vi "Initialize FakedArray.vi"(4 "User events":T8, 6 "Color":T7=9868950, 7 "ToMoreSpecific":T9, 8 "error in (no error)":errorcluster, 9 "Data":T10, 10 "Cluster Refnum":refnum<vi>, 11 "Data in":T1={"Class"={"Ants"=refnum, "Layer"=refnum, "Templates"=refnum, "Icon"=refnum, "Glyph"=refnum, "Settings"=refnum, "Tools"=refnum}, "Ref"={"Add Layer"=refnum, "Remove Layer"=refnum, "Line Text"=[], "Body Text Spec"=refnum, "DNL_Font"=refnum, "glyph path str"=refnum, "templates path str"=refnum, "Arrow Up"=refnum, "Arrow Down"=refnum, "IE VI Ref"=refnum, "Glyphs tree"=refnum, "Templates tree"=refnum, "Layer Icon Text"=refnum, "Layer Template"=refnum, "Clipboard"=refnum, "BW icon in"=refnum, "Color icon in"=refnum, "Layer Clust"=refnum, "Body Text"=refnum, "DNL_Framework Templates"=refnum, "Search Templates"=refnum, "TextMarker"=refnum, "Tab Control"=refnum, "Search Glyphs"=refnum, "Line Color"=refnum, "DNL_Glyphs []"=refnum, "Fill Color"=refnum, "Tools"=refnum, "Glyphs tree"=refnum, "Icon"=refnum, "Preview"=refnum, "Ants"=refnum, "Terminals"=refnum, "menu reference"=refnum, "LayerNames"=[], "GlyphLoadAnimation"=refnum, "TemplateLoadAnimation"=refnum, "refreshGlyphs"=refnum, "refreshTemplates"=refnum}, "Support"={"AntsRect"={"left"=0, "top"=0, "right"=0, "bottom"=0}, "Mouse Move Coords"={"Horizontal"=0, "Vertical"=0}, "Mouse Down Coords"={"Horizontal"=0, "Vertical"=0}, "Temp Coord"={"Horizontal"=0, "Vertical"=0}, "Action"=enum."Default", "Edge Color"=4914962, "Fill Color"=16860, "Mouse Down?"=FALSE, "Draft Mode?"=FALSE, "Temp Icon"=bytes[3102], "CTRL Pressed"=FALSE, "Move Selection?"=FALSE, "AntsRect Orig"={"left"=0, "top"=0, "right"=0, "bottom"=0}, "Text"="", "TM Set?"=FALSE, "Mouse inside icon?"=FALSE, "Tool (old value)"=0, "Pencil Move Color"=0, "Swap Colors?"=FALSE, "Shift pressed?"=FALSE}}) -> (0 "error out":errorcluster, 3 "Data out":T1={"Class"={"Ants"=refnum, "Layer"=refnum, "Templates"=refnum, "Icon"=refnum, "Glyph"=refnum, "Settings"=refnum, "Tools"=refnum}, "Ref"={"Add Layer"=refnum, "Remove Layer"=refnum, "Line Text"=[], "Body Text Spec"=refnum, "DNL_Font"=refnum, "glyph path str"=refnum, "templates path str"=refnum, "Arrow Up"=refnum, "Arrow Down"=refnum, "IE VI Ref"=refnum, "Glyphs tree"=refnum, "Templates tree"=refnum, "Layer Icon Text"=refnum, "Layer Template"=refnum, "Clipboard"=refnum, "BW icon in"=refnum, "Color icon in"=refnum, "Layer Clust"=refnum, "Body Text"=refnum, "DNL_Framework Templates"=refnum, "Search Templates"=refnum, "TextMarker"=refnum, "Tab Control"=refnum, "Search Glyphs"=refnum, "Line Color"=refnum, "DNL_Glyphs []"=refnum, "Fill Color"=refnum, "Tools"=refnum, "Glyphs tree"=refnum, "Icon"=refnum, "Preview"=refnum, "Ants"=refnum, "Terminals"=refnum, "menu reference"=refnum, "LayerNames"=[], "GlyphLoadAnimation"=refnum, "TemplateLoadAnimation"=refnum, "refreshGlyphs"=refnum, "refreshTemplates"=refnum}, "Support"={"AntsRect"={"left"=0, "top"=0, "right"=0, "bottom"=0}, "Mouse Move Coords"={"Horizontal"=0, "Vertical"=0}, "Mouse Down Coords"={"Horizontal"=0, "Vertical"=0}, "Temp Coord"={"Horizontal"=0, "Vertical"=0}, "Action"=enum."Default", "Edge Color"=4914962, "Fill Color"=16860, "Mouse Down?"=FALSE, "Draft Mode?"=FALSE, "Temp Icon"=bytes[3102], "CTRL Pressed"=FALSE, "Move Selection?"=FALSE, "AntsRect Orig"={"left"=0, "top"=0, "right"=0, "bottom"=0}, "Text"="", "TM Set?"=FALSE, "Mouse inside icon?"=FALSE, "Tool (old value)"=0, "Pencil Move Color"=0, "Swap Colors?"=FALSE, "Shift pressed?"=FALSE}})   [LabVIEW 2021, in "FakedArray.lvclass"]
uses:
  FakedArray.lvclass
  Controls/ToMoreSpecific_Faked2DArray.ctl
  vi.lib/LabVIEW Icon API/lv_icon/Controls/IEColor.ctl
  Controls/IE Data.ctl
  Ants/Ants.lvclass
  vi.lib/LabVIEW Icon API/lv_icon/Classes/Icon/Icon.lvclass
  Icon Library/Glyph.lvclass
  Settings/Settings.lvclass
  Tools/Tools Paint.lvclass
  Controls/IE Classes.ctl
  Controls/References Cluster.ctl
  Controls/SupportClass.ctl
  <vilib>/Utility/miscctls.llb/LVPoint32TypeDef.ctl
  Controls/SupportClass_Action.ctl
  FakedArray.lvclass/FakedArray.ctl
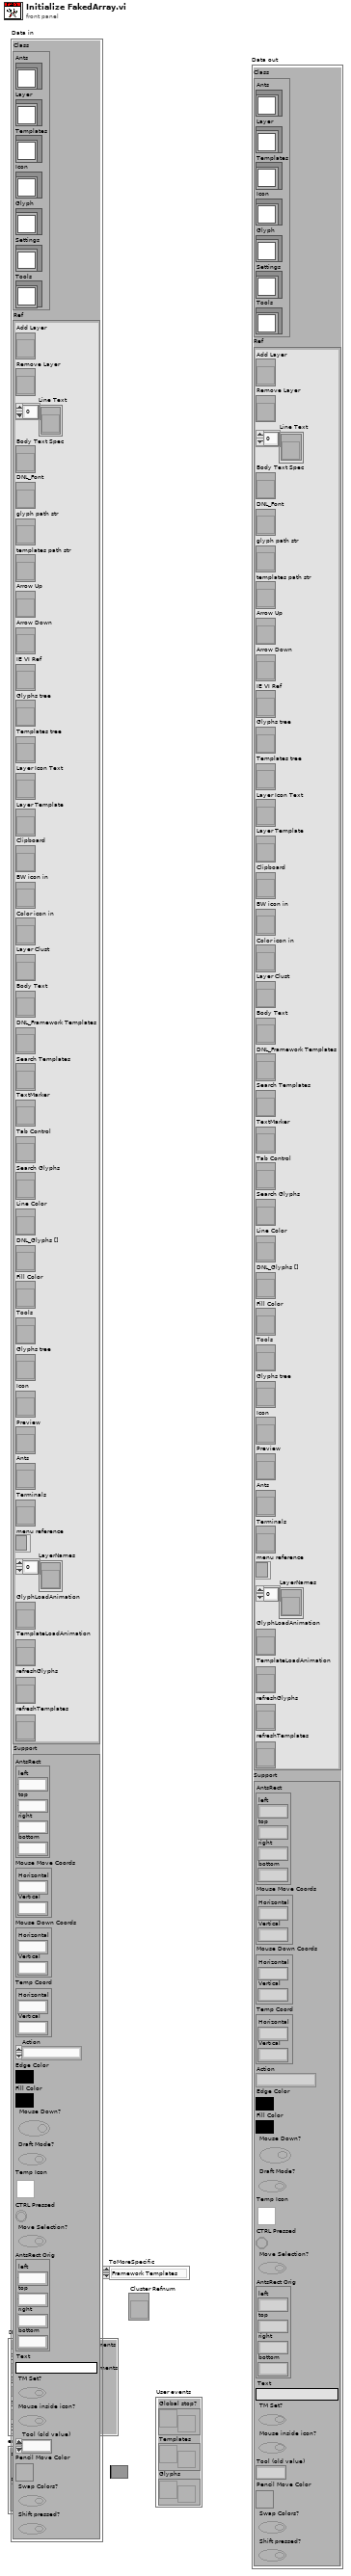
[diagram p1: front panel]
types:
  T1 = typedef "IE Data.ctl" = cluster{"Class":T2, "Ref":T3, "Support":T4}
  T2 = typedef "IE Classes.ctl" = cluster{"Ants":refnum<class "Ants.lvclass">, "Layer":refnum<class "FakedArray.lvclass">, "Templates":refnum<class "FakedArray.lvclass">, "Icon":refnum<class "Icon.lvclass">, "Glyph":refnum<class "Glyph.lvclass">, "Settings":refnum<class "Settings.lvclass">, "Tools":refnum<class "Tools Paint.lvclass">}
  T3 = typedef "References Cluster.ctl" = cluster{"Add Layer":refnum<vi>, "Remove Layer":refnum<vi>, "Line Text":refnum<vi>[], "Body Text Spec":refnum<vi>, "DNL_Font":refnum<vi>, "glyph path str":refnum<vi>, "templates path str":refnum<vi>, "Arrow Up":refnum<vi>, "Arrow Down":refnum<vi>, "IE VI Ref":refnum<vi>, "Glyphs tree":refnum<vi>, "Templates tree":refnum<vi>, "Layer Icon Text":refnum<vi>, "Layer Template":refnum<vi>, "Clipboard":refnum<vi>, "BW icon in":refnum<vi>, "Color icon in":refnum<vi>, "Layer Clust":refnum<vi>, "Body Text":refnum<vi>, "DNL_Framework Templates":refnum<vi>, "Search Templates":refnum<vi>, "TextMarker":refnum<vi>, "Tab Control":refnum<vi>, "Search Glyphs":refnum<vi>, "Line Color":refnum<vi>, "DNL_Glyphs []":refnum<vi>, "Fill Color":refnum<vi>, "Tools":refnum<vi>, "Glyphs tree":refnum<vi>, "Icon":refnum<vi>, "Preview":refnum<vi>, "Ants":refnum<vi>, "Terminals":refnum<vi>, "menu reference":refnum<k9>, "LayerNames":refnum<vi>[], "GlyphLoadAnimation":refnum<vi>, "TemplateLoadAnimation":refnum<vi>, "refreshGlyphs":refnum<vi>, "refreshTemplates":refnum<vi>}
  T4 = typedef "SupportClass.ctl" = cluster{"AntsRect":cluster{"left":i16, "top":i16, "right":i16, "bottom":i16}, "Mouse Move Coords":T5, "Mouse Down Coords":T5, "Temp Coord":T5, "Action":T6, "Edge Color":T7, "Fill Color":T7, "Mouse Down?":bool, "Draft Mode?":bool, "Temp Icon":picture, "CTRL Pressed":bool, "Move Selection?":bool, "AntsRect Orig":cluster{"left":i16, "top":i16, "right":i16, "bottom":i16}, "Text":string, "TM Set?":bool, "Mouse inside icon?":bool, "Tool (old value)":u32, "Pencil Move Color":u32, "Swap Colors?":bool, "Shift pressed?":bool}
  T5 = typedef "LVPoint32TypeDef.ctl" = cluster{"Horizontal":i32, "Vertical":i32}
  T6 = typedef "SupportClass_Action.ctl" = enum16{"Default", "Move Selection", "Glyph Library", "Tool"}
  T7 = typedef "IEColor.ctl" = u32
  T8 = cluster{"Global stop?":refnum<user-event>, "Templates":refnum<user-event>, "Glyphs":refnum<user-event>}
  T9 = typedef "ToMoreSpecific_Faked2DArray.ctl" = enum16{"Framework Templates", "Layer List"}
  T10 = cluster{"Minimum # of selected elements":u32, "Maximum # of selected elements":u32, "# Rows":u32, "# Cols":u32}
  T11 = typedef "Path&Icon.ctl" = cluster{"Rectangle":cluster{"left":i16, "top":i16, "right":i16, "bottom":i16}, "Path":path, "Image":picture, "Filter":string, "FileName":string}
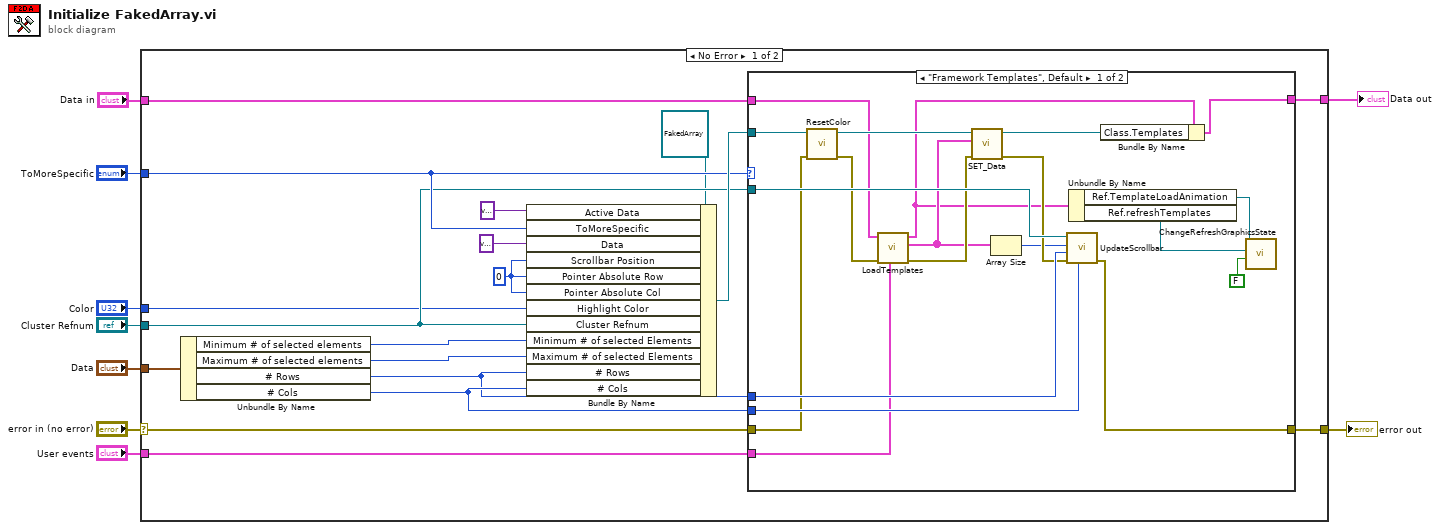
[diagram p0: block diagram]
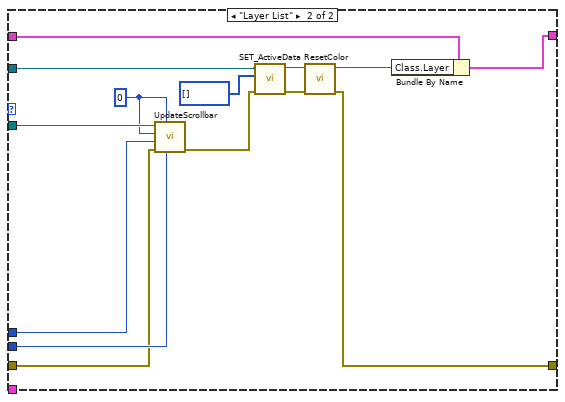
[diagram p2: hidden frame]
diagram:
  n1 = case shown="No Error" "error in (no error)" {
    selector: "error in (no error)" -> [w13 w63]
    tunnel: [w23 w63] -> w4
    tunnel: "Cluster Refnum" -> [w19 _]
    tunnel: "Data" -> [w27 _]
    tunnel: "ToMoreSpecific" -> [w20 _]
    tunnel: "Color" -> [w16 _]
    tunnel: "User events" -> [w12 _]
    tunnel: "Data in" -> [w11 w62]
    tunnel: [w10 w62] -> w1
    frame No Error {
      w22 = u32 0 ("Pointer Absolute Row")
      n2 = Unbundle By Name(w27) -> ("Minimum # of selected elements"=w26:u32, "Maximum # of selected elements"=w25:u32, "# Rows"=w17:u32, "# Cols"=w18:u32)
      n3 = Bundle By Name(cluster=refnum<class "FakedArray.lvclass"> refnum ("FakedArray in"), "Active Data"=variant, "ToMoreSpecific"=w20, "Data"=variant, "Scrollbar Position"=w22, "Pointer Absolute Row"=w22, "Pointer Absolute Col"=w22, "Highlight Color"=w16, "Cluster Refnum"=w19, "Minimum # of selected Elements"=w26, "Maximum # of selected Elements"=w25, "# Rows"=w17, "# Cols"=w18) -> (w24:refnum<class "FakedArray.lvclass">)
      n4 = case shown="\"Framework Templates\", Default" w20 {
        tunnel: w24 -> [w44 w56]
        tunnel: [w34 w48] -> w23
        tunnel: w19 -> [w47 w61]
        tunnel: w17 -> [w45 w59]
        tunnel: w18 -> [w46 w60]
        tunnel: w13 -> [w42 w57]
        tunnel: w12 -> [w37 _]
        tunnel: w11 -> [w32 w51]
        tunnel: [w35 w49] -> w10
        frame "Framework Templates", Default {
          n5 = call "ResetColor.vi"("error in (no error)"=w42, "FakedArray in"=w44) -> ("error out"=w40:errorcluster, "FakedArray out"=w43:refnum<class "FakedArray.lvclass">)  [unwired: 8 out]
          n6 = call "LoadTemplates.vi"("User events"=w37, "error in (no error)"=w40, "Data in"=w32) -> ("error out"=w39:errorcluster, "Glyphs[]"=w33:T11[], "Data out"=w30:T1)  [unwired: 6 out]
          n7 = call-dynamic "SET_Data.vi"("error in (no error)"=w39, "Data"=w33, "FakedArray in"=w43) -> ("error out"=w41:errorcluster, "FakedArray out"=w36:refnum<class "FakedArray.lvclass">)  [unwired: 7 out]
          n8 = Array Size(array=w33) -> (size(s)=w38:i32)
          n9 = call "UpdateScrollbar.vi"("# Cols"=w46, "error in"=w41, "#Rows"=w45, "# Elements"=w38, "Cluster Refnum"=w47) -> ("error out"=w34:errorcluster)  [unwired: 1 in, 5 out]
          n10 = Unbundle By Name(w30) -> ("Ref.TemplateLoadAnimation"=w29:refnum<vi>, "Ref.refreshTemplates"=w28:refnum<vi>)
          n11 = Bundle By Name(cluster=w30, "Class.Templates"=w36) -> (w35:T1)
          n12 = call "ChangeRefreshGraphicsState.vi"("refreshing?"=FALSE, "button ref"=w28, "animatedDecoration ref"=w29) -> ()  [unwired: 8 in, 1 out]
        }
        frame "Layer List" {
          w58 = 0 ("# Elements")
          n13 = call "UpdateScrollbar.vi"("# Cols"=w60, "Value Scrollbar"=w58, "error in"=w57, "#Rows"=w59, "# Elements"=w58, "Cluster Refnum"=w61) -> ("error out"=w55:errorcluster)  [unwired: 5 out]
          n14 = call-dynamic "SET_ActiveData.vi"("error in (no error)"=w55, "Active Data"=i32[] [], "FakedArray.lvclass in"=w56) -> ("error out"=w53:errorcluster, "FakedArray.lvclass out"=w52:refnum<class "FakedArray.lvclass">)  [unwired: 7 out]
          n15 = call "ResetColor.vi"("error in (no error)"=w53, "FakedArray in"=w52) -> ("error out"=w48:errorcluster, "FakedArray out"=w50:refnum<class "FakedArray.lvclass">)  [unwired: 8 out]
          n16 = Bundle By Name(cluster=w51, "Class.Layer"=w50) -> (w49:T1)
        }
      }
    }
    frame Error {
    }
  }
  "error out" <- w4
  "Data out" <- w1
